vi "Generate script array elements.vi"(3 "Script in":T2[](array[typedef]) {"Carousel" items=["0", "1", "2", "3", "4", "5", "6"]; "Positioners [mm|°]" min=-1.0 max=330.0; "Tau [ms]" min=0.002 max=10000.0; "Wait [min]" min=0.0 max=3000.0; "Tmp [K]" min=0.0 max=350.0; "Mod_A [G]" min=0.0 max=100.0; "Mod_F [kHz]" min=0.1 max=150.0}, 4 "Generator options":T1={"Tmp step [K]"=0.0, "Angle step [°]"=[], "Freq step [GHz]"=0.0, "Append"=TRUE, "Iterate"=0}, 5 "Prototype line":T2={"Start"=0.0, "Start Caption"="Start [T]", "End"=0.0, "End Caption"="End [T]", "Sweep"=0.0, "Sweep caption"="Rate [mT/s]", "Constant"=0.0, "Constant caption"="Freq [GHz]", "Mod_F [kHz]"=0.0, "Mod_A [G]"=0.0, "Tau [ms]"=0.0, "Positioners [mm|°]"=[-1.0], "Tmp [K]"=50.0, "Wait [min]"=0.0, "Carousel"=-1, "Comment"="", "Auto-mod"=TRUE, "Execute"=FALSE} {"Carousel" items=["0", "1", "2", "3", "4", "5", "6"]; "Positioners [mm|°]" min=-1.0 max=330.0; "Tau [ms]" min=0.002 max=10000.0; "Wait [min]" min=0.0 max=3000.0; "Tmp [K]" min=0.0 max=350.0; "Mod_A [G]" min=0.0 max=100.0; "Mod_F [kHz]" min=0.1 max=150.0}) -> (1 "Script out":T2[](array[typedef]) {"Carousel" items=["0", "1", "2", "3", "4", "5", "6"]; "Positioners [mm|°]" min=-1.0 max=330.0; "Tau [ms]" min=0.002 max=10000.0; "Wait [min]" min=0.0 max=3000.0; "Tmp [K]" min=0.0 max=350.0; "Mod_A [G]" min=0.0 max=100.0; "Mod_F [kHz]" min=0.1 max=150.0})   [LabVIEW 2022 SP3]
uses:
  Datatypes/script polymorh line.ctl
panel:
  # "Inputs"
  # "Outputs"
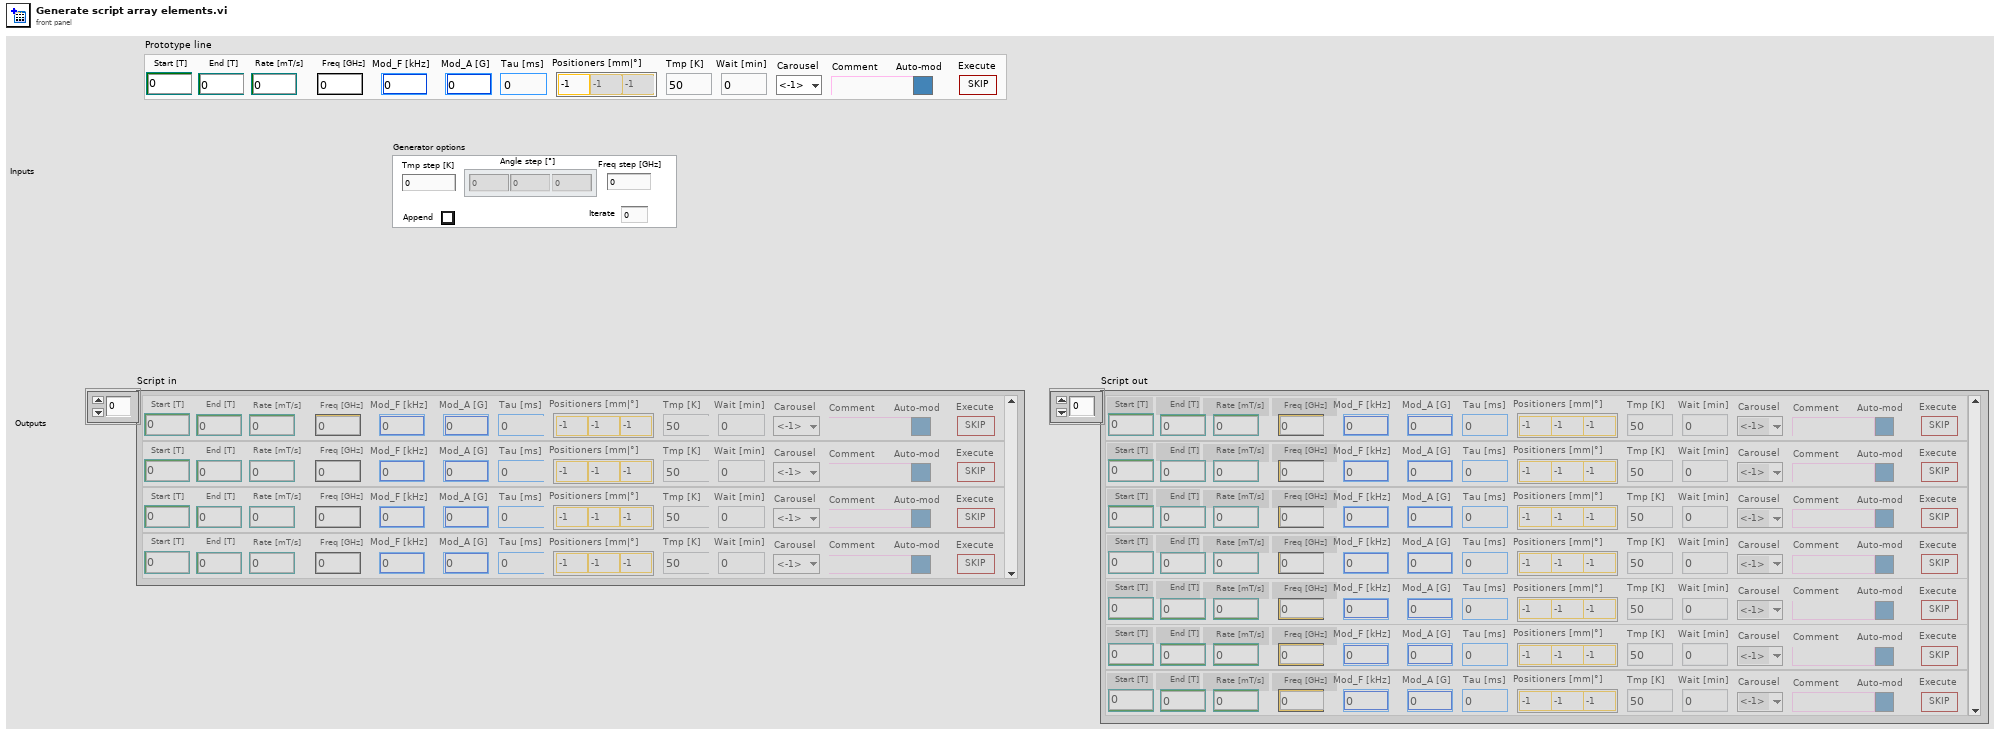
[diagram p1: front panel]
types:
  T1 = cluster{"Tmp step [K]":dbl, "Angle step [°]":dbl[], "Freq step [GHz]":dbl, "Append":bool, "Iterate":u16}
  T2 = typedef "script polymorh line.ctl" = cluster{"Start":dbl, "Start Caption":string, "End":dbl, "End Caption":string, "Sweep":dbl, "Sweep caption":string, "Constant":dbl, "Constant caption":string, "Mod_F [kHz]":dbl, "Mod_A [G]":dbl, "Tau [ms]":dbl, "Positioners [mm|°]":dbl[], "Tmp [K]":dbl, "Wait [min]":dbl, "Carousel":i8, "Comment":string, "Auto-mod":bool, "Execute":bool}
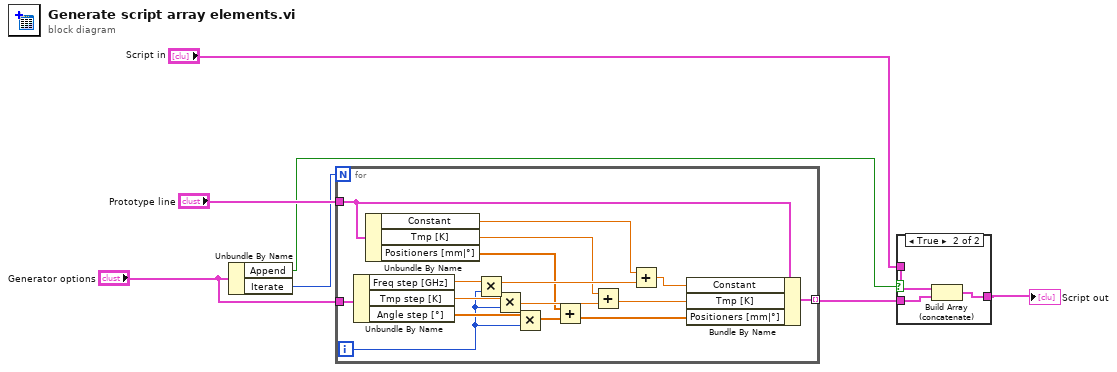
[diagram p0: block diagram]
diagram:
  n1 = Unbundle By Name("Generator options") -> ("Append"=w3:bool, "Iterate"=w5:u16)
  n2 = for {
    N: w5 -> [_]
    tunnel: "Generator options" -> [w22]
    tunnel: [w23] -> w7 mode=indexing
    tunnel: "Prototype line" -> [w14]
    i -> [w15]
    n3 = Unbundle By Name(w22) -> ("Freq step [GHz]"=w21:dbl, "Tmp step [K]"=w20:dbl, "Angle step [°]"=w19:dbl[])
    n4 = Unbundle By Name(w14) -> ("Constant"=w12:dbl, "Tmp [K]"=w8:dbl, "Positioners [mm|°]"=w9:dbl[])
    n5 = Multiply(x=w21, y=w15) -> (x*y=w18:dbl)
    n6 = Multiply(x=w20, y=w15) -> (x*y=w17:dbl)
    n7 = Multiply(x=w19, y=w15) -> (x*y=w16:dbl[])
    n8 = Add(x=w9, y=w16) -> (x+y=w10:dbl[])
    n9 = Add(x=w8, y=w17) -> (x+y=w11:dbl)
    n10 = Add(x=w12, y=w18) -> (x+y=w13:dbl)
    n11 = Bundle By Name(cluster=w14, "Constant"=w13, "Tmp [K]"=w11, "Positioners [mm|°]"=w10) -> (w23:T2)
  }
  n12 = case shown="True" w3 {
    tunnel: w7 -> [w24 w27]
    tunnel: [w24 w26] -> w2
    tunnel: "Script in" -> [_ w25]
    frame False {
    }
    frame True {
      n13 = Build Array (concatenate)(w25, w27) -> (w26:T2[])
    }
  }
  "Script out" <- w2
